vi "Generate.vi"(8 "error in (no error)":errorcluster, 10 "X Center":i32, 11 "object in":refnum<class "Piece of Bricks.lvclass">) -> (0 "error out":errorcluster, 3 "object out":refnum<class "Piece of Bricks.lvclass">)   [LabVIEW 2017, in "Piece of Bricks.lvclass"]
uses:
  Piece of Bricks.lvclass
  Piece of Bricks.lvclass/Piece of Bricks.ctl
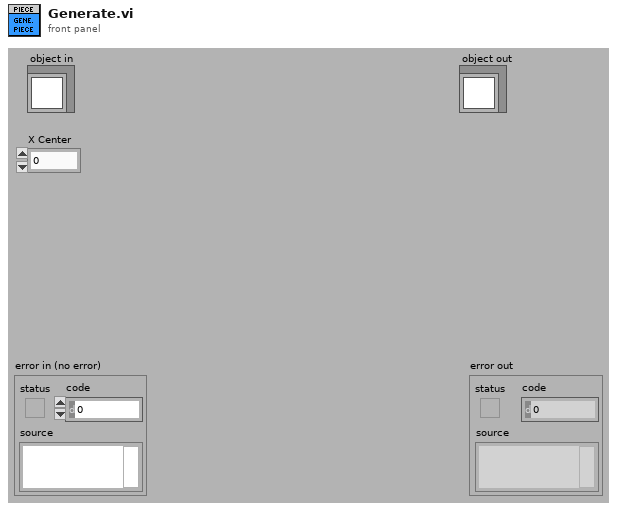
[diagram p1: front panel]
types:
  T1 = typedef "Pieces Geometry Names.ctl" = enum16{"I", "O", "T", "L", "J", "Z", "S"}
  T2 = typedef "Pieces Description.ctl" = T3[]
  T3 = typedef "Piece Description.ctl" = cluster{"Pieces Geometry Names":T1, "Piece Color":u32, "Coordinates":T4[], "X Offset":i32, "Y Offset":i32, "Rotation State":T5}
  T4 = typedef "Coordinates.ctl" = cluster{"X":i32, "Y":i32}
  T5 = typedef "Rotation State.ctl" = enum16{"0", "90", "180", "270"}
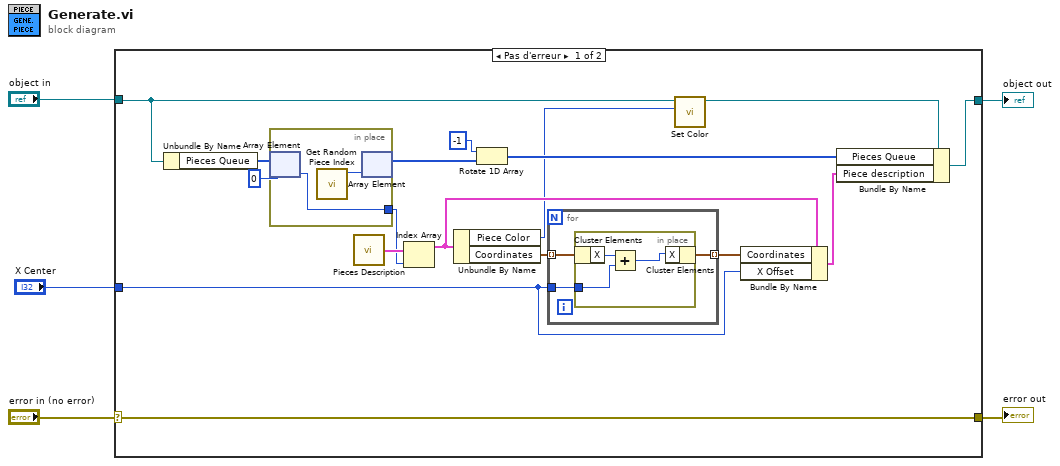
[diagram p0: block diagram]
diagram:
  n1 = case shown="Pas d'erreur" "error in (no error)" {
    selector: "error in (no error)" -> [w22 w32]
    tunnel: [w22 w32] -> w4
    tunnel: [w21 w31] -> w2
    tunnel: "object in" -> [w8 w31]
    tunnel: "X Center" -> [w9 _]
    frame No Error {
      n2 = Unbundle By Name(w8) -> ("Pieces Queue"=w20:T1[])
      n3 = in-place {
        in-place-border: [w29] -> w15
        n4 = in-place-array #1(w20, 0) -> (w29:T1)
        n5 = call "Get Random Piece Index.vi"() -> ("Piece index"=w30:u16)  [unwired: 10 in, 1 out]
        n6 = in-place-array #1(w30) -> (w19:T1[])  [unwired: 1 out]
      }
      n7 = call "Pieces Description.vi"() -> ("Pieces Description"=w16:T2)  [unwired: 1 in]
      n8 = Index Array(array=w16, index=w15) -> (element=w12:T3)
      n9 = Unbundle By Name(w12) -> ("Piece Color"=w6:u32, "Coordinates"=w14:T4[])
      n10 = Rotate 1D Array(1:w19, 2:-1 ("n")) -> (0:w18:T1[])
      n11 = for {
        tunnel: w14 -> [w25] mode=indexing
        tunnel: w9 -> [w24]
        tunnel: [w23] -> w11 mode=indexing
        n12 = in-place {
          in-place-border: w24 -> [w27]
          n13 = in-place-cluster #2(w25) -> ("X"=w28:i32)
          n14 = Add(x=w28, y=w27) -> (x+y=w26:i32)
          n15 = in-place-cluster #2("X"=w26) -> (w23:T4)
        }
      }
      n16 = call-dynamic "Set Color.vi"("Color"=w6, "object in"=w8) -> ("object out"=w7:refnum<class "Piece of Bricks.lvclass">)  [unwired: 8 in, 1 out]
      n17 = Bundle By Name(cluster=w12, "Coordinates"=w11, "X Offset"=w9) -> (w10:T3)
      n18 = Bundle By Name(cluster=w7, "Pieces Queue"=w18, "Piece description"=w10) -> (w21:refnum<class "Piece of Bricks.lvclass">)
    }
    frame Error {
    }
  }
  "error out" <- w4
  "object out" <- w2
